vi "SV TDMS Write Scalar (1 Ch).vi"(0 "tdms file":refnum<k34>, 1 "write channel properties (T)":bool=TRUE, 5 "group name in (Feature)":string="Feature", 7 "channel name in (Channel0)":string="Channel0", 9 "value in":dbl, 11 "error in":errorcluster, 12 "scalar info in":T1={"scalar function type"=10, "scalar function subtype"=19, " x-dimension"=0} {"scalar function type" items=["Speed"=3, "Ratio"=6, "Count"=7, "-"=9, "Level"=10, "-"=19, "None"=98]; "scalar function subtype" items=["Value"=19, "DC"=11, "AC"=12, "RMS^2"=13, "RMS"=14, "Peak"=15, "Peak to peak"=16, "-"=20, "Phase"=33, "-"=90, "None"=98, "Unknown"=99]; "x-dimension" items=["Time (s)"=0, "Frequency-CB (Hz)"=1, "Frequency-CPB (Hz)"=1248, "Frequency-Arbitrary (Hz)"=2357, "Quefrency (s)"=2, "Revolutions (rev)"=3, "Order"=4, "Speed (RPM)"=11, "Speed (rad/s)"=21, "Critical Band"=31, "Critical Band Rate (Bark)"=32, "None"=98, "Index"=65535]}, 13 "Y-unit label (\"\")":string) -> (4 "tdms file out":refnum<k34>, 6 "group name out":string, 8 "channel name out":string, 15 "error out":errorcluster)   [LabVIEW 2017]
doc: "Writes data to the specified .tdms file in a format specific to the polymorphic instance. Wire data to the <B>scaled signal [EU]</B> input to determine the polymorphic instance to use or manually select the instance."
uses:
  <vilib>/addons/_NISVFA/_Shared subVIs/Controls/NI Scalar Function Info.ctl
  <vilib>/addons/_NISVFA/_Shared subVIs/Controls/svc_X-Axis Units.ctl
  <vilib>/addons/_NISVFA/_Shared subVIs/Controls/LV Datatypes.ctl
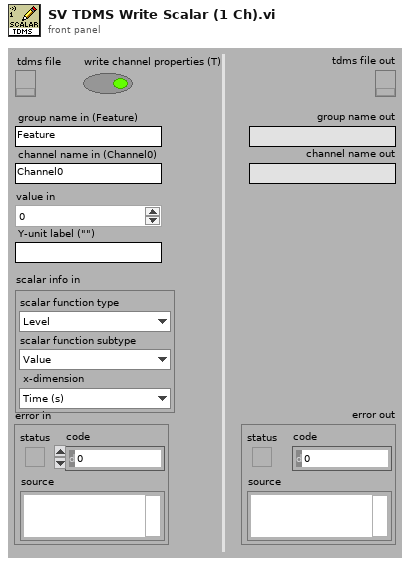
[diagram p1: front panel]
types:
  T1 = typedef "NI Scalar Function Info.ctl" = cluster{"scalar function type":u16, "scalar function subtype":u16, " x-dimension":T2}
  T2 = typedef "svc_X-Axis Units.ctl" = u16
  T3 = typedef "LV Datatypes.ctl" = i32
  T4 = typedef "svc_Unit Info.ctl" = cluster{"X-axis label":string, "X-unit string":string, "Y-axis label":string, "Y-unit string":string}
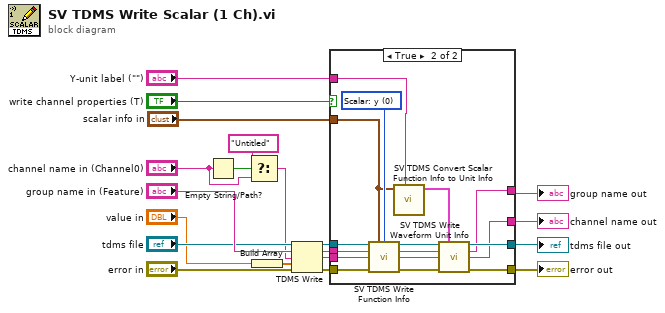
[diagram p0: block diagram]
diagram:
  n1 = Empty String/Path?(string/path="channel name in (Channel0)") -> (empty?=w5:bool)
  n2 = Select(t="Untitled", s=w5, f="channel name in (Channel0)") -> (s? t:f=w2:string)
  n3 = Build Array("value in") -> (w7:dbl[])
  n4 = TDMS Write(0:"tdms file", 5:"group name in (Feature)", 7:w2, 9:w7, 11:"error in") -> (4:w11:refnum<k34>, 6:w10:string, 8:w9:string, 15:w8:errorcluster)  [unwired: 1 in]
  n5 = case shown="True" "write channel properties (T)" {
    tunnel: [w22 w36] -> w20
    tunnel: w11 -> [w22 w35]
    tunnel: w10 -> [w24 w34]
    tunnel: w9 -> [w23 w33]
    tunnel: w8 -> [w21 w32]
    tunnel: [w21 w31] -> w19
    tunnel: [w23 w30] -> w15
    tunnel: [w24 w29] -> w16
    tunnel: "Y-unit label (\"\")" -> [_ w25]
    tunnel: "scalar info in" -> [_ w27]
    frame False {
    }
    frame True {
      w28 = T3 0 items=["String"=-2, "Boolean"=-1, "Scalar: y"=0, "Array: Y"=1, "Waveform: t0, dt, Y, variant"=2, "Cluster: x0, dx, Y"=3, "Cluster: X, Y"=4, "Waterfall"=5, "Colormap"=6] ("LabVIEW datatype")
      n6 = call <vilib>:"SV TDMS Write Function Info.vi"("tdms file in"=w35, "function info"=w27, "LabVIEW datatype"=w28, "group name"=w34, "channel name"=w33, "error in (no error)"=w32) -> ("tdms file out"=w40:refnum<k34>, "group name out"=w39:string, "channel name out"=w38:string, "error out"=w37:errorcluster)  [unwired: 6 in]
      n7 = call <vilib>:"SV TDMS Convert Scalar Function Info to Unit Info.vi"("Y-unit string override"=w25, "scalar info in"=w27) -> ("unit info"=w26:T4)  [unwired: 9 in]
      n8 = call <vilib>:"SV TDMS Write Waveform Unit Info.vi"("tdms file"=w40, "unit info"=w26, "group name"=w39, "channel name"=w38, "error in (no error)"=w37) -> ("tdms file out"=w36:refnum<k34>, "group name out"=w29:string, "channel name out"=w30:string, "error out"=w31:errorcluster)  [unwired: 7 in]
    }
  }
  "tdms file out" <- w20
  "error out" <- w19
  "channel name out" <- w15
  "group name out" <- w16
